vi "Get Trigger Source.vi"(8 "error in (no error)":errorcluster, 11 "Camera in":refnum<class "Camera.lvclass">) -> (0 "error out":errorcluster, 2 "Trigger Source":string, 3 "Camera":refnum<class "Camera.lvclass">)   [LabVIEW 2020, in "Camera.lvclass"]
uses:
  Camera.lvclass
  Camera.lvclass/Camera.ctl
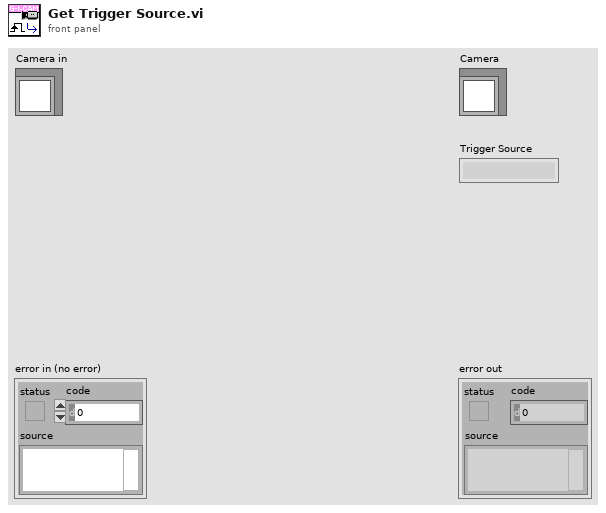
[diagram p1: front panel]
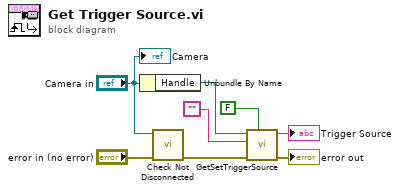
[diagram p0: block diagram]
diagram:
  n1 = Unbundle By Name("Camera in") -> ("Handle"=w5:refnum<data-value>)
  n2 = call "Check Not Disconnected.vi"("error in (no error)"="error in (no error)", "Camera in"="Camera in") -> ("error out"=w2:errorcluster)  [unwired: 9 in]
  n3 = call "GetSetTriggerSource.vi"("Set"=FALSE, "error in (no error)"=w2, "Source"="", "Data Value Reference in"=w5) -> ("error out"=→"error out":errorcluster, "Source"=→"Trigger Source":string)  [unwired: 6 in]
  "Camera" <- "Camera in"
